vi "GetVISAInstrSettings.vi"(8 "error in (no error)":errorcluster, 10 "Param In":string, 11 "Get Settings from GPIB Addrs List":string) -> (0 "error out":errorcluster, 3 "Param Out":string)   [LabVIEW 2015]
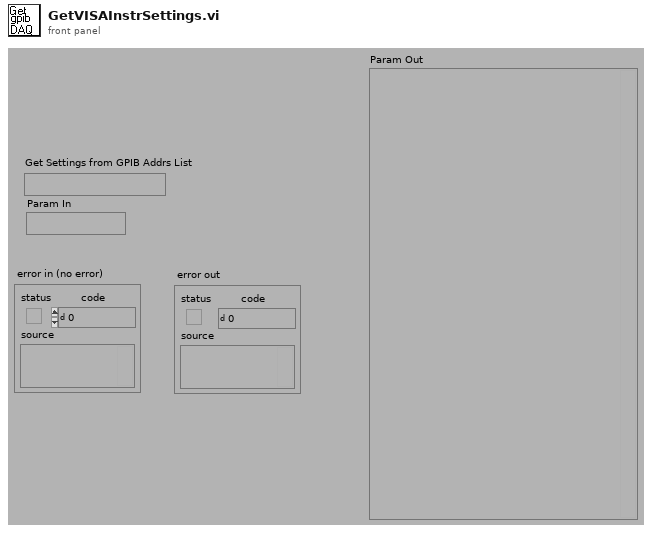
[diagram p1: front panel]
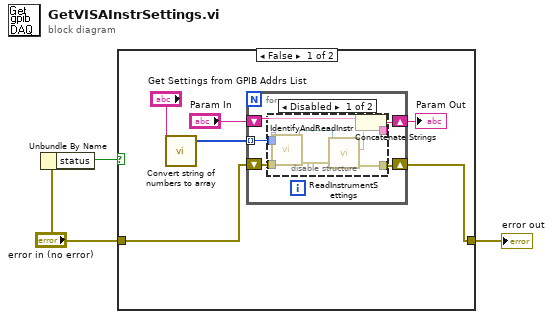
[diagram p0: block diagram]
diagram:
  n1 = Unbundle By Name("error in (no error)") -> ("status"=w1:bool)
  n2 = case shown="False" w1 {
    tunnel: "error in (no error)" -> [w8 w23]
    tunnel: [w4 w23] -> w2
    frame False {
      n3 = call "Convert string of numbers to array.vi"("#'s string"="Get Settings from GPIB Addrs List") -> ("#'s Array"=w9:i16[])  [unwired: 4 in]
      n4 = for {
        tunnel: w9 -> [w13] mode=indexing
        shift-right: [w10] -> w4
        shift-left: w8 -> [w14]
        shift-right: [w12] -> w6
        shift-left: "Param In" -> [w11]
        n5 = disable-structure shown="Disabled" {
          disable-tunnel: w14 -> [w22 _]
          disable-tunnel: w13 -> [w21 _]
          disable-tunnel: [w20 _] -> w12
          disable-tunnel: w11 -> [w19 _]
          disable-tunnel: [w16 _] -> w10
          frame Disabled {
            n6 = call "IdentifyAndReadInstr.vi"("error in (no error)"=w22, "VISA Resource Name"=w21) -> ("error out"=w18:errorcluster, "VISA Resource Name Out"=w17:refnum<visa-resource-name>)  [unwired: 6 in, 2 out]
            n7 = call "ReadInstrumentSettings.vi"("error in (no error)"=w18, "Instrument type/address"=w17) -> ("error out"=w16:errorcluster, "Parameters"=w15:string)  [unwired: 7 in, 1 out]
            n8 = Concatenate Strings(w19, w15) -> (w20:string)
          }
          frame Enabled {
          }
        }
      }
      "Param Out" <- w6
    }
    frame True {
    }
  }
  "error out" <- w2
